vi "初始化队列.vi"(8 "error in (no error)":errorcluster) -> (0 "error out":errorcluster, 2 "输出簇":T1)   [LabVIEW 2015]
uses:
  <vilib>/vision/Image Controls.llb/IMAQ Image.ctl
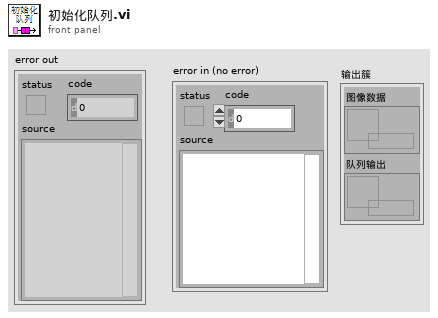
[diagram p1: front panel]
types:
  T1 = cluster{"图像数据":refnum<queue>, "队列输出":refnum<queue>}
  T2 = typedef "IMAQ Image.ctl" = refnum<image>
  T3 = cluster{"周长":dbl, "面积":dbl, "3D":u8[], "灰度图像":T2, "3D view":T2, "滤波":T2, "边缘检测":T2, "3D图像":T2, "质心坐标X":sgl, "质心坐标Y":sgl, "第一点y值，x=0":dbl, "第二点y值，x=639":dbl, "第一点x值，y=0":dbl, "第二点x值，y=479":dbl, "短轴半径um":dbl, "长轴半径um":dbl, "长轴长度":dbl, "短轴长度":dbl, "短轴原曲线":dbl[], "长轴拟合":dbl[], "纵轴拟合":dbl[], "横轴拟合":dbl[], "长轴原曲线":dbl[], "纵轴原曲线":dbl[], "横轴原曲线":dbl[], "短轴拟合":dbl[], "位置":dbl, "触发":bool, "初始化后退":bool, "初始化前进":bool}
  T4 = cluster{"图像数据":refnum<queue>, "手动取点":refnum<queue>}
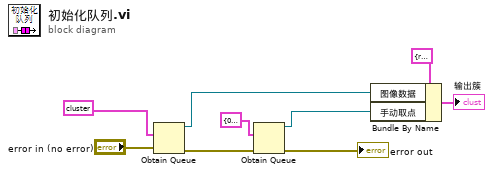
[diagram p0: block diagram]
diagram:
  n1 = Obtain Queue(element data type=T3 {"周长"=0.0, "面积"=0.0, "3D"=[], "灰度图像"=refnum, "3D view"=refnum, "滤波"=refnum, "边缘检测"=refnum, "3D图像"=refnum, "质心坐标X"=0.0, "质心坐标Y"=0.0, "第一点y值，x=0"=0.0, "第二点y值，x=639"=0.0, "第一点x值，y=0"=0.0, "第二点x值，y=479"=0.0, "短轴半径um"=0.0, "长轴半径um"=0.0, "长轴长度"=0.0, "短轴长度"=0.0, "短轴原曲线"=[], "长轴拟合"=[], "纵轴拟合"=[], "横轴拟合"=[], "长轴原曲线"=[], "纵轴原曲线"=[], "横轴原曲线"=[], "短轴拟合"=[], "位置"=0.0, "触发"=FALSE, "初始化后退"=FALSE, "初始化前进"=FALSE}, error in (no error)="error in (no error)") -> (queue out=w7:refnum<queue>, error out=w5:errorcluster)  [unwired: 3 in, 1 out]
  n2 = Obtain Queue(element data type=cluster{"手动取点y":i32, "手动取点x":i32, "是否手动取点":bool} {"手动取点y"=0, "手动取点x"=0, "是否手动取点"=TRUE} ("手动取点"), error in (no error)=w5) -> (queue out=w1:refnum<queue>, error out=→"error out":errorcluster)  [unwired: 3 in, 1 out]
  n3 = Bundle By Name(cluster=T4 {"图像数据"=refnum, "手动取点"=refnum} ("Queue Refs"), "图像数据"=w7, "手动取点"=w1) -> (→"输出簇":T4)
